vi "Map.vi"(8 "地图比例":dbl(slide)=3.0 min=3.0 max=18.0 step=1.0 scale=6.0..18.0, 10 "纬度":string, 11 "经度":string) -> (2 "BaiduMapURL":string)   [LabVIEW 2018]
panel:
  out "最新经纬度":string
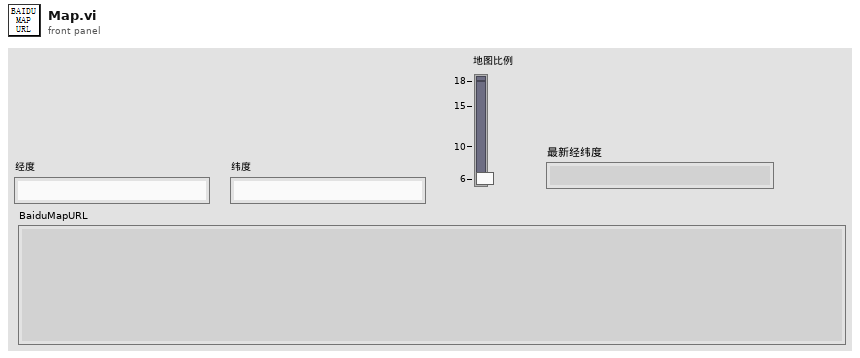
[diagram p1: front panel]
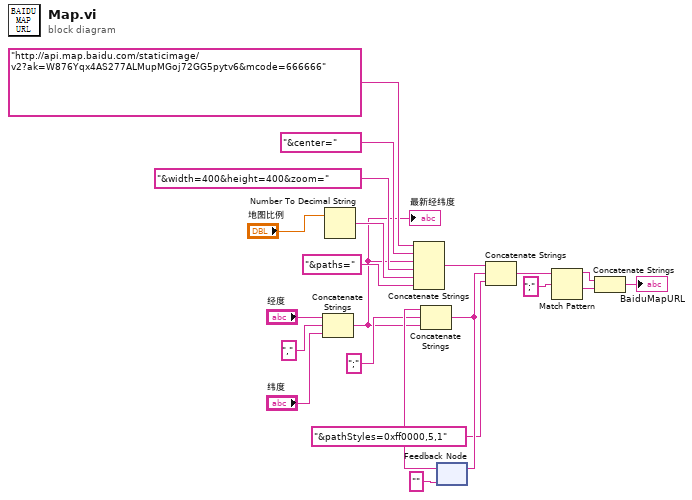
[diagram p0: block diagram]
diagram:
  n1 = Concatenate Strings("经度", ",", "纬度") -> (w11:string)
  "最新经纬度" <- w11
  n2 = Number To Decimal String(number="地图比例") -> (decimal integer string=w14:string)  [unwired: 1 in]
  n3 = Concatenate Strings("http://api.map.baidu.com/staticimage/v2?ak=W876Yqx4AS277ALMupMGoj72GG5pytv6&mcode=666666", "&center=" ("字符串"), w11, "&width=400&height=400&zoom=" ("字符串"), w14, "&paths=") -> (w10:string)
  n4 = feedback #1("") -> (w13:string)
  n5 = Concatenate Strings(w13, ";" ("字符串"), w11) -> (w9:string)
  n6 = feedback-in #1(w9) -> ()
  n7 = Concatenate Strings(w10, w9, "&pathStyles=0xff0000,5,1" ("字符串")) -> (w4:string)
  n8 = Match Pattern(string=w4, regular expression=";" ("正则表达式")) -> (before substring=w6:string, after substring=w5:string)  [unwired: 1 in, 2 out]
  n9 = Concatenate Strings(w6, w5) -> (→"BaiduMapURL":string)
